vi "Search Array Example 01.vi"() -> ()   [LabVIEW 2011]
uses:
  <userlib>/_OpenG.lib/array/array.llb/Search 1D Array (I8)__ogtk.vi
panel:
  out "Indices for All 2s after Index 1":i32[](array[numeric])
  out "Indices for All 3s":i32[](array[numeric])
  in  "Array":i8[](array[numeric])=[2, 4, 2, 7, 9, 1, 3, 5, 3, 2, 8, 0]
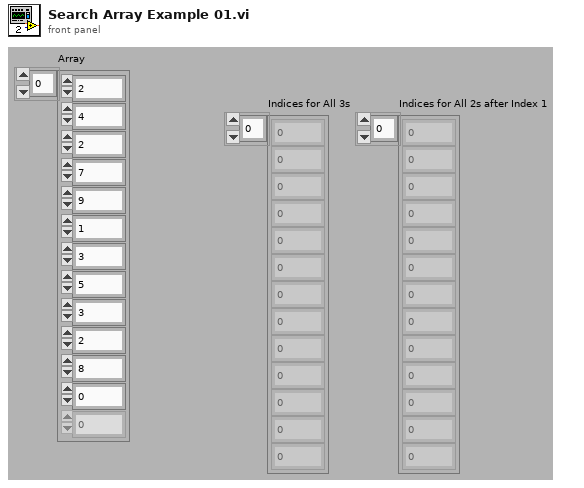
[diagram p1: front panel]
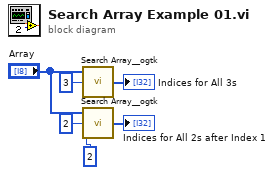
[diagram p0: block diagram]
diagram:
  n1 = call-poly <userlib>:"Search Array__ogtk.vi"("Array"="Array", "Element Data"=i8 3) -> ("Indices of Elements"=→"Indices for All 3s":i32[])  [unwired: 7 in]
  n2 = call-poly <userlib>:"Search Array__ogtk.vi"("Array"="Array", "Element Data"=i8 2, "Start Index (0)"=2) -> ("Indices of Elements"=→"Indices for All 2s after Index 1":i32[])  [unwired: 6 in]
